vi "setLogFilePath.vi"(8 "error in (no error)":errorcluster, 11 "Protocol_Generic out 2":refnum<class "Protocol_Logging.lvclass">) -> (0 "error out":errorcluster, 3 "Protocol_Generic out":refnum<class "Protocol_Logging.lvclass">)   [LabVIEW 2011, in "Protocol_Logging.lvclass"]
uses:
  Protocol_Logging.lvclass
  Protocol_Logging.lvclass/Protocol_Logging.ctl
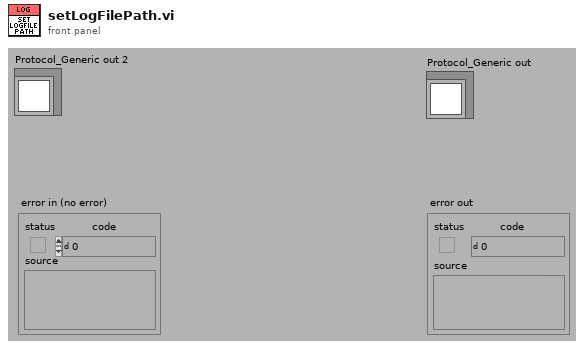
[diagram p1: front panel]
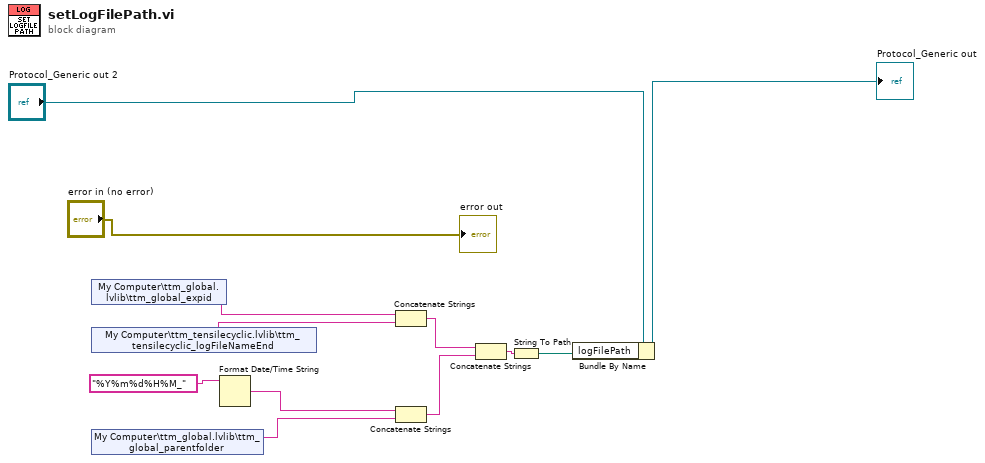
[diagram p0: block diagram]
diagram:
  n1 = shared-variable "My Computer\\ttm_global.lvlib\\ttm_global_expid"() -> (w3:string)  [unwired: 1 in, 1 out]
  n2 = shared-variable "My Computer\\ttm_tensilecyclic.lvlib\\ttm_tensilecyclic_logFileNameEnd"() -> (w2:string)  [unwired: 1 in, 1 out]
  n3 = shared-variable "My Computer\\ttm_global.lvlib\\ttm_global_parentfolder"() -> (w9:string)  [unwired: 1 in, 1 out]
  n4 = Format Date/Time String(time format string (%c)="%Y%m%d%H%M_") -> (date/time string=w7:string)  [unwired: 2 in]
  n5 = Concatenate Strings(w3, w2) -> (w10:string)
  n6 = Concatenate Strings(w7, w9) -> (w8:string)
  n7 = Concatenate Strings(w10, w8) -> (w11:string)
  n8 = String To Path(string=w11) -> (path=w12:path)
  n9 = Bundle By Name(cluster="Protocol_Generic out 2", "logFilePath"=w12) -> (→"Protocol_Generic out":refnum<class "Protocol_Logging.lvclass">)
  "error out" <- "error in (no error)"
